vi "Image Pack Control.vi"(9 "Numeric in":u32, 10 "input valid":bool, 11 "PMT1_signal":u16) -> (1 "Numeric out":u32, 2 "packer out":T1, 3 "output valid?":bool)   [LabVIEW 2015]
uses:
  DRAM data index.ctl
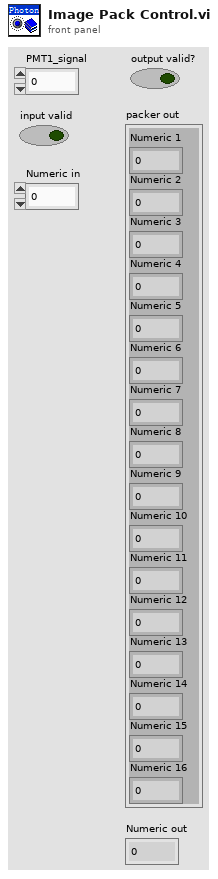
[diagram p1: front panel]
types:
  T1 = cluster{"Numeric 1":u32, "Numeric 2":u32, "Numeric 3":u32, "Numeric 4":u32, "Numeric 5":u32, "Numeric 6":u32, "Numeric 7":u32, "Numeric 8":u32, "Numeric 9":u32, "Numeric 10":u32, "Numeric 11":u32, "Numeric 12":u32, "Numeric 13":u32, "Numeric 14":u32, "Numeric 15":u32, "Numeric 16":u32}
  T2 = typedef "DRAM data index.ctl" = enum16{"Numeric 1", "Numeric 2", "Numeric 3", "Numeric 4", "Numeric 5", "Numeric 6", "Numeric 7", "Numeric 8", "Numeric 9", "Numeric 10", "Numeric 11", "Numeric 12", "Numeric 13", "Numeric 14", "Numeric 15", "Numeric 16"}
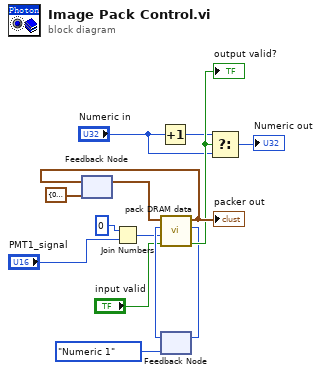
[diagram p0: block diagram]
diagram:
  n1 = feedback #1(T1 {"Numeric 1"=0, "Numeric 2"=0, "Numeric 3"=0, "Numeric 4"=0, "Numeric 5"=0, "Numeric 6"=0, "Numeric 7"=0, "Numeric 8"=0, "Numeric 9"=0, "Numeric 10"=0, "Numeric 11"=0, "Numeric 12"=0, "Numeric 13"=0, "Numeric 14"=0, "Numeric 15"=0, "Numeric 16"=0} ("packer out")) -> (w13:T1)
  n2 = Join Numbers(hi=u16 0, lo="PMT1_signal") -> ((hi.lo)=w4:u32)
  n3 = Increment(x="Numeric in") -> (x+1=w9:u32)
  n4 = feedback #2(DRAM_data_index."Numeric 1" ("DRAM Index out")) -> (w6:T2)
  n5 = call "pack DRAM data.vi"("input valid?"="input valid", "data to be packed"=w4, "DRAM Index in"=w6, "packer in"=w13) -> ("output valid?"=w12:bool, "DRAM Index out"=w5:T2, "packer out"=w14:T1)  [unwired: 5 in]
  "packer out" <- w14
  "output valid?" <- w12
  n6 = feedback-in #1(w14) -> ()
  n7 = feedback-in #2(w5) -> ()
  n8 = Select(t=w9, s=w12, f="Numeric in") -> (s? t:f=→"Numeric out":u32)
